vi "waitForMagnet.vi"(6 "Axis":T1, 8 "error in (no error)":errorcluster, 9 "Tolerance (T)":dbl, 10 "Setpoint (T)":dbl, 11 "Instrument.Cryostat in":refnum<class "Instrument.Cryostat.lvclass">) -> (0 "error out":errorcluster, 3 "Instrument.Cryostat out":refnum<class "Instrument.Cryostat.lvclass">)   [LabVIEW 2019, in "Instrument.Cryostat.lvclass"]
uses:
  Instrument.Cryostat.lvclass
  Typedefs/Magnet Axis--Enum.ctl
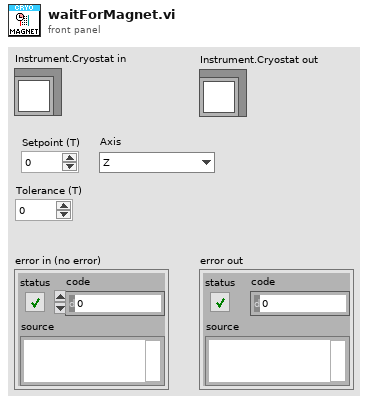
[diagram p1: front panel]
types:
  T1 = typedef "Instrument.Cryostat.lvclass/Magnet Axis--Enum.ctl" = enum16{"Z", "X", "Y"}
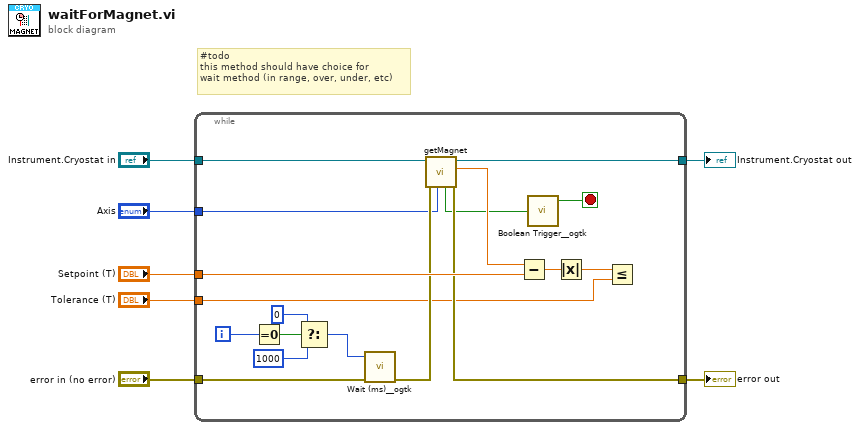
[diagram p0: block diagram]
diagram:
  # "#todo\nthis method should have choice for\nwait method (in range, over, under, etc)"
  n1 = while {
    tunnel: "Setpoint (T)" -> [w23]
    tunnel: "error in (no error)" -> [w19]
    tunnel: [w21] -> w7
    tunnel: "Instrument.Cryostat in" -> [w18]
    tunnel: [w17] -> w3
    tunnel: "Axis" -> [w16]
    tunnel: "Tolerance (T)" -> [w15]
    i -> [w12]
    stop <- w13 stop-if-true
    n2 = Equal To 0?(x=w12) -> (x = 0?=w11:bool)
    n3 = Select(t=u32 0, s=w11, f=u32 1000 ("milliseconds to wait")) -> (s? t:f=w8:u32)
    n4 = call <userlib>:"Wait (ms)__ogtk.vi"("error in (no error)"=w19, "milliseconds to wait"=w8) -> ("error out"=w22:errorcluster)  [unwired: 8 in, 1 out]
    n5 = call-dynamic "getMagnet.vi"("Axis"=w16, "error in (no error)"=w22, "Instrument.Cryostat in"=w18) -> ("error out"=w21:errorcluster, "B Field (T)"=w20:dbl, "Instrument.Cryostat out"=w17:refnum<class "Instrument.Cryostat.lvclass">, "Finished?"=w14:bool)  [unwired: 4 in, 1 out]
    n6 = Subtract(x=w20, y=w23) -> (x-y=w25:dbl)
    n7 = call <userlib>:"Boolean Trigger__ogtk.vi"("Boolean Input"=w14) -> ("Rising Edge"=w13:bool)  [unwired: 1 in, 1 out]
    n8 = Absolute Value(x=w25) -> (abs(x)=w24:dbl)
    n9 = Less Or Equal?(x=w24, y=w15) -> ()  [unwired: 1 out]
  }
  "Instrument.Cryostat out" <- w3
  "error out" <- w7
